vi "UpdateRequestRaw.vi"(7 "Data to update":T1, 8 "error in":errorcluster, 9 "data":variant, 10 "RequestID":string) -> (0 "error out":errorcluster)   [LabVIEW 2015, in "DatabaseApi.lvlib"]
uses:
  DatabaseApi.lvlib
  TypeDef/Request/RequestsTableColumnNamesRing.ctl
  TypeDef/Request/RequestsTableDbTableName.ctl
  <vilib>/addons/database/Connection.llb/DB Tools Open Connec (Path).vi
  <vilib>/addons/database/NI_Database_API.lvlib
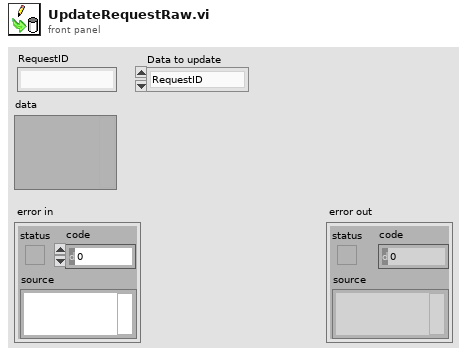
[diagram p1: front panel]
types:
  T1 = typedef "DatabaseApi.lvlib/RequestsTableColumnNamesRing.ctl" = enum16{"RequestID", "PersonnelType", "StartTime", "StartName", "AckTime", "AckName", "FulfilledTime", "FulfilledName", "Description", "Room Number", "Request Type", "Alarm"}
  T2 = typedef "DatabaseApi.lvlib/RequestsTableDbTableName.ctl" = string
  T3 = typedef "NI_Database_API.lvlib/Conn ObjectReference.ctl" = refnum<k1>
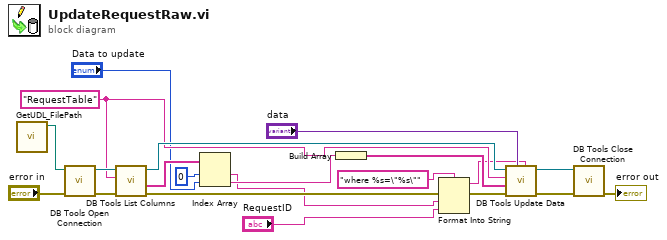
[diagram p0: block diagram]
diagram:
  w11 = T2 "RequestTable" ("table")
  n1 = call "GetUDL_FilePath.vi"() -> ("UDL file path"=w21:path)  [unwired: 11 in]
  n2 = call-poly <vilib>:"DB Tools Open Connection.vi"("error in (no error)"="error in", "connection information"=w21) -> ("error out"=w18:errorcluster, "connection reference"=w14:T3)  [unwired: 6 in]
  n3 = call <vilib>:"DB Tools List Columns.vi"("error in (no error)"=w18, "table"=w11, "connection reference"=w14) -> ("error out"=w15:errorcluster, "columns"=w12:string[], "connection reference out"=w13:T3)  [unwired: 1 in, 1 out]
  n4 = Index Array(array=w12, index #1=0 ("index"), index #2="Data to update") -> (element #1=w7:string, element #2=w10:string)
  n5 = Build Array(w10) -> (w4:string[])
  n6 = Format Into String(format string="where %s=\"%s\"", error in=w15, w7, "RequestID") -> (resulting string=w1:string, error out=w2:errorcluster)  [unwired: 1 in]
  n7 = call <vilib>:"DB Tools Update Data.vi"("condition"=w1, "data"="data", "error in (no error)"=w2, "columns"=w4, "table"=w11, "connection reference"=w13) -> ("error out"=w17:errorcluster, "connection reference out"=w16:T3)  [unwired: 4 in]
  n8 = call <vilib>:"DB Tools Close Connection.vi"("error in (no error)"=w17, "connection reference"=w16) -> ("error out"=→"error out":errorcluster)  [unwired: 5 in]
